vi "DAQ_Assistant_Ref_Signal.vi"(8 "device name":tag="Dev2", 9 "stop (F)":bool, 10 "rate":dbl=1000.0, 11 "number of samples":i32=100) -> (2 "data 2":dynamicdata(graph) caption="data")   [LabVIEW 2012]
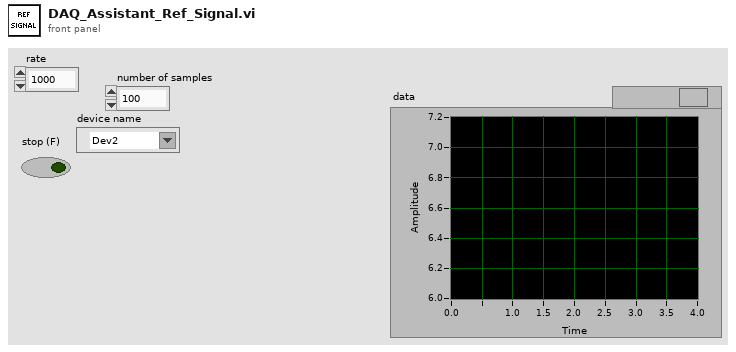
[diagram p1: front panel]
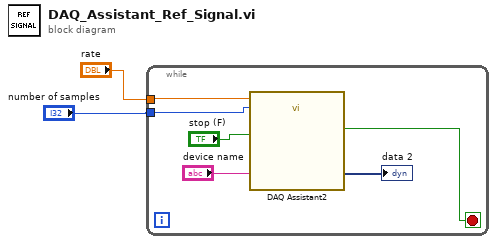
[diagram p0: block diagram]
diagram:
  n1 = while {
    tunnel: "rate" -> [w6]
    tunnel: "number of samples" -> [w4]
    stop <- w5 stop-if-true
    n2 = call "DAQ Assistant2"("rate"=w6, "number of samples"=w4, "stop (F)"="stop (F)", "device name"="device name") -> ("data"=→"data 2":dynamicdata, "stopped"=w5:bool)  [unwired: 12 in, 2 out]
  }
